vi "[FPGA] PI FXPT Simple (FPGA, Use outside SCTL).vi"(0 "Setpoint":sgl, 1 "lower limit":sgl=-32768.0, 2 "upper limit":sgl=32768.0, 5 "Process Variable":sgl, 7 "Enable":bool=TRUE, 9 "Kp":sgl=1.0 step=0.125, 11 "Ki*Ts":sgl, 12 "Reset Value":sgl format="%#_31g", 13 "Reset":bool) -> (4 "Output":sgl format="%.2f")   [LabVIEW 2015]
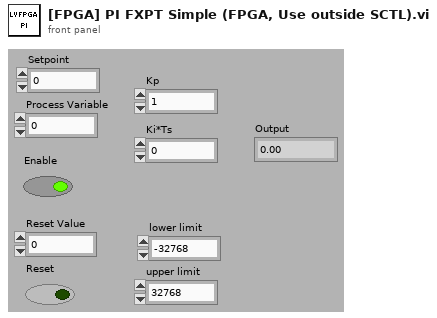
[diagram p1: front panel]
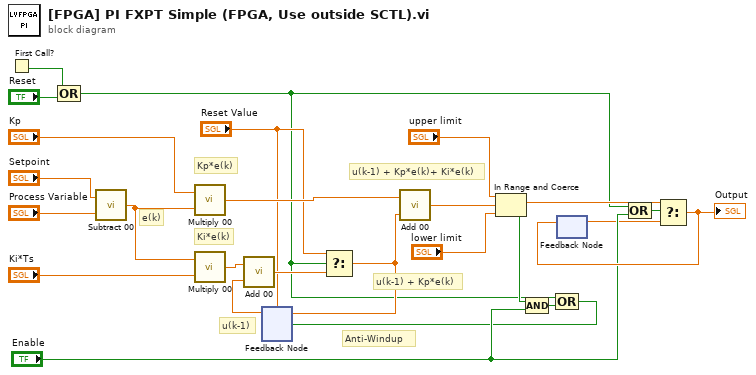
[diagram p0: block diagram]
diagram:
  # "u(k-1) + Kp*e(k)"
  # "Anti-Windup"
  # "u(k-1)"
  # "Kp*e(k)"
  # "Ki*e(k)"
  # "e(k)"
  # "u(k-1) + Kp*e(k)+ Ki*e(k)"
  n1 = First Call?() -> (First Call?: T/F=w1:bool)
  n2 = Compound Arithmetic op=OR(w1, "Reset") -> (w2:bool)
  n3 = call "Subtract 00.vi"("y"="Process Variable", "x"="Setpoint") -> ("x*y"=w19:sgl)
  n4 = call "Multiply 00.vi"("y"=w19, "x"="Kp") -> ("x*y"=w23:sgl)
  n5 = call "Multiply 00.vi"("y"="Ki*Ts", "x"=w19) -> ("x*y"=w21:sgl)
  n6 = feedback #1("Reset Value") -> (w4:sgl)
  n7 = call "Add 00.vi"("y"=w4, "x"=w21) -> ("x+y"=w17:sgl)
  n8 = Select(t="Reset Value", s=w2, f=w17) -> (s? t:f=w5:sgl)
  n9 = call "Add 00.vi"("y"=w5, "x"=w23) -> ("x+y"=w20:sgl)
  n10 = In Range and Coerce(upper limit="upper limit", x=w20, lower limit="lower limit") -> (coerced(x)=w14:sgl, In Range?=w10:bool)
  n11 = Compound Arithmetic op=AND(w10, "Enable") -> (w8:bool)
  n12 = Compound Arithmetic op=OR(w2, w8) -> (w6:bool)
  n13 = feedback-in #1(w5, w6) -> ()
  n14 = feedback #2() -> (w3:sgl)  [unwired: 1 in]
  n15 = Compound Arithmetic op=OR(w2, "Enable") -> (w12:bool)
  n16 = Select(t=w14, s=w12, f=w3) -> (s? t:f=w13:sgl)
  "Output" <- w13
  n17 = feedback-in #2(w13) -> ()
